vi "Temp.vi"() -> ()   [LabVIEW 2025]
uses:
  user32.dll
panel:
  out "x":u32
  out "return type 2":i32
  out "error out":errorcluster
  in  "error in (no error)":errorcluster
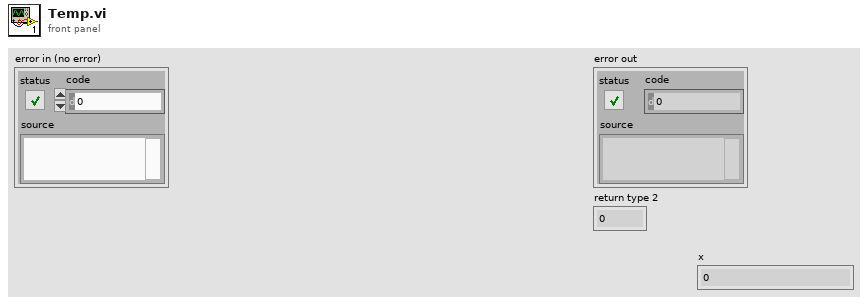
[diagram p1: front panel]
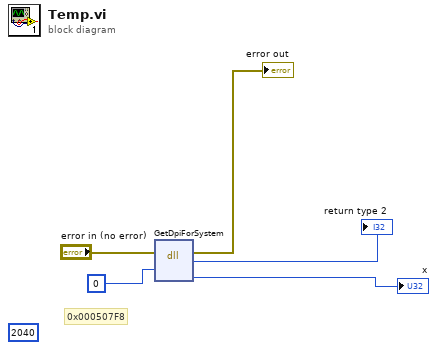
[diagram p0: block diagram]
diagram:
  (unwired) i16 2040 ("x")
  # "0x000507F8"
  n1 = dll-call lib="User32.dll" fn="GetDpiForSystem" ("user32.dll:GetCursorPos")(error in="error in (no error)", "hWnd"=i64 0 ("x")) -> (error out=→"error out":errorcluster, "return type"=→"return type 2":i32, "DPI"=→"x":u32)  [unwired: 2 in, 3 out]
